vi "ReportPart.vi"(6 "试验项目":enum32{"手柄锁紧力", "手柄开启力", "手柄推拉力", "手柄保持力"}(ring), 8 "error in":errorcluster, 9 "索引IN":i32, 10 "合格":T1, 11 "report in":refnum<class "NI_report.lvclass">) -> (0 "error out 2":errorcluster caption="error out", 2 "索引OUT":i32, 3 "report out":refnum<class "NI_report.lvclass">)   [LabVIEW 2020]
uses:
  <vilib>/Utility/NIReport.llb/NI_report.lvclass
  OK.ctl
  <vilib>/Utility/NIReport.llb/image depth.ctl
  <vilib>/addons/_office/_exclsub.llb/font.ctl
  Global_Variable/A180648.vi
  <vilib>/Utility/NIReport.llb/Append Report Text (str wrap).vi
  Global_Variable/Global.vi
  <vilib>/addons/_office/word.llb/Word Easy Table (str).vi
  <vilib>/Utility/NIReport.llb/NI_ReportGenerationCore.lvlib
  <vilib>/addons/_office/NI_ReportGenerationToolkit.lvlib
  <vilib>/Utility/NIReport.llb/Word/NI_Word.lvclass
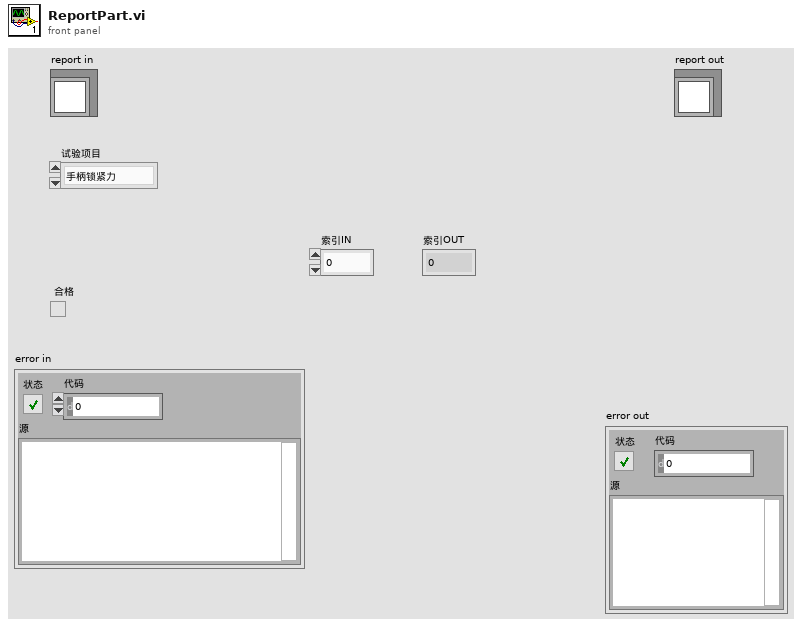
[diagram p1: front panel]
types:
  T1 = typedef "OK.ctl" = bool
  T2 = cluster{"Charset (-1)":i16, "Weight (-1)":i16, "Name":string, "Size":string}
  T3 = cluster{"Italic":enum16{"Italic Unchanged", "Italic On", "Italic Off"}, "Strike Through":enum16{"Strike Through Unchanged", "Strike Through On", "Strike Through Off"}, "Underline":enum16{"Underline Unchanged", "Underline On", "Underline Off"}, "Bold":enum16{"Bold Unchanged", "Bold On", "Bold Off"}}
  T4 = typedef "NI_ReportGenerationToolkit.lvlib/font.ctl" = cluster{"font name":string, "font size":dbl, "bold":u16, "italic":u16, "underline":u16, "strike through":u16, "font color":u32}
  T5 = typedef "NI_ReportGenerationCore.lvlib/image depth.ctl" = u16
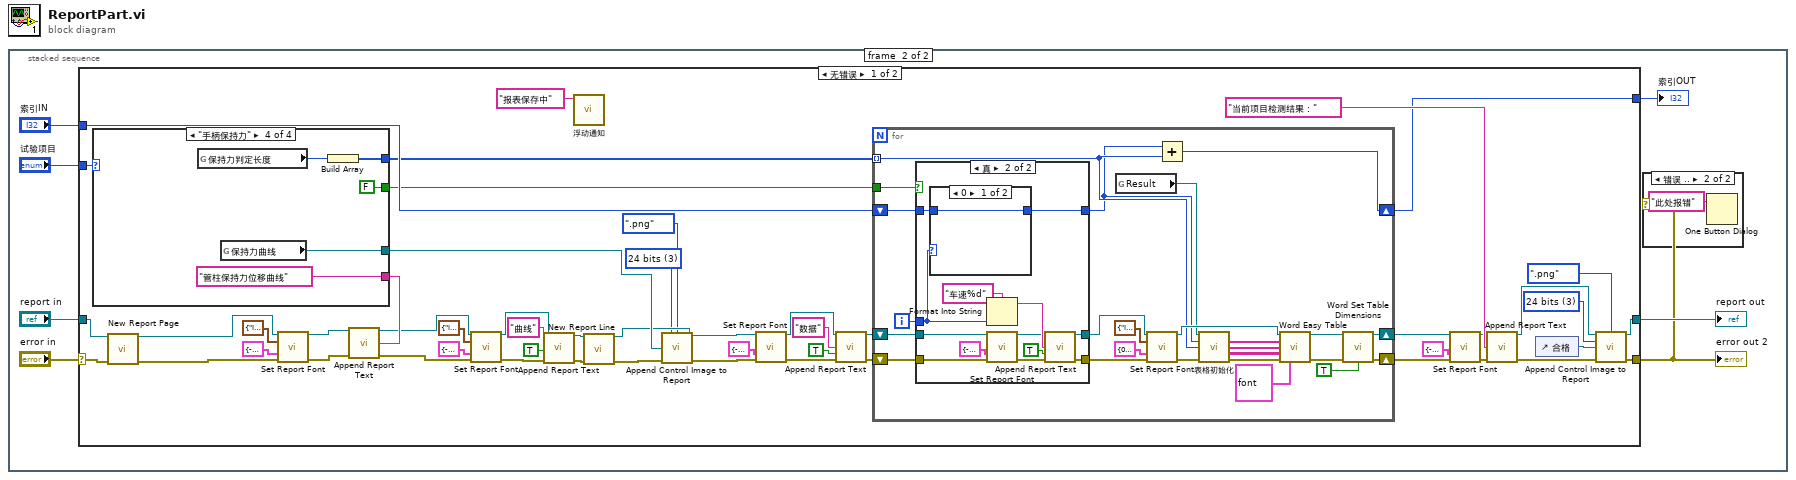
[diagram p0: block diagram]
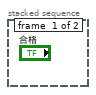
[diagram p2: hidden frame]
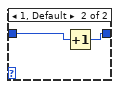
[diagram p5: hidden frame]
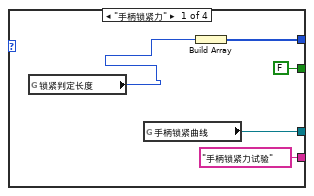
[diagram p6: hidden frame]
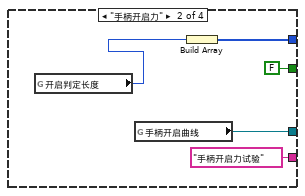
[diagram p7: hidden frame]
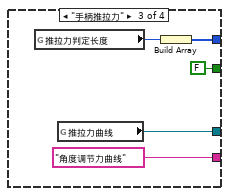
[diagram p8: hidden frame]
diagram:
  n1 = stacked-sequence {
    frame #0 {
    }
    frame #1 {
      n2 = case shown="无错误" "error in" {
        selector: "error in" -> [w53 w127]
        tunnel: [w48 w127] -> w1
        tunnel: "索引IN" -> [w20 w126]
        tunnel: "试验项目" -> [w23 _]
        tunnel: [w17 w126] -> w4
        tunnel: [w22 w125] -> w3
        tunnel: "report in" -> [w21 w125]
        frame No Error {
          w36 = T5 3 items=["B&W", "4 bits", "8 bits", "24 bits"] ("image depth")
          w46 = T5 3 items=["B&W", "4 bits", "8 bits", "24 bits"] ("image depth")
          n3 = case shown="\"手柄保持力\"" w23 {
            tunnel: [w109 w114 w119 w124] -> w39
            tunnel: ["手柄锁紧力试验" ("text") "手柄开启力试验" ("text") "角度调节力曲线" ("text") "管柱保持力位移曲线" ("text")] -> w57
            tunnel: [w107 w112 w115 w120] -> w19
            tunnel: [FALSE FALSE FALSE FALSE] -> w16
            frame "手柄锁紧力" {
              n4 = global read "判定参数.vi" "锁紧判定长度"() -> (w105:i32)
              n5 = global read "A180648.vi" "手柄锁紧曲线"() -> (w109:refnum<vi>)
              n6 = Build Array(w105) -> (w107:i32[])
            }
            frame "手柄开启力" {
              n7 = global read "判定参数.vi" "开启判定长度"() -> (w110:i32)
              n8 = global read "A180648.vi" "手柄开启曲线"() -> (w114:refnum<vi>)
              n9 = Build Array(w110) -> (w112:i32[])
            }
            frame "手柄推拉力" {
              n10 = global read "判定参数.vi" "推拉力判定长度"() -> (w117:i32)
              n11 = global read "A180648.vi" "推拉力曲线"() -> (w119:refnum<vi>)
              n12 = Build Array(w117) -> (w115:i32[])
            }
            frame "手柄保持力" {
              n13 = global read "判定参数.vi" "保持力判定长度"() -> (w122:i32)
              n14 = global read "A180648.vi" "保持力曲线"() -> (w124:refnum<vi>)
              n15 = Build Array(w122) -> (w120:i32[])
            }
          }
          n16 = call-dynamic "New Report Page.vi"("report in"=w21, "error in (no error)"=w53) -> ("report out"=w51:refnum<class "NI_report.lvclass">, "error out"=w52:errorcluster)  [unwired: 12 in]
          n17 = call-dynamic "Set Report Font.vi"("report in"=w51, "text options"=T3 {"Italic"=enum."Italic Unchanged", "Strike Through"=enum."Strike Through Unchanged", "Underline"=enum."Underline Unchanged", "Bold"=enum."Bold On"}, "font settings"=T2 {"Charset (-1)"=-1, "Weight (-1)"=-1, "Name"="楷体", "Size"="16 "}, "error in (no error)"=w52) -> ("report out"=w60:refnum<class "NI_report.lvclass">, "error out"=w59:errorcluster)  [unwired: 9 in, 1 out]
          n18 = call-poly <vilib>:"Append Report Text.vi"("report in"=w60, "text"=w57, "error in (no error)"=w59) -> ("report out"=w55:refnum<class "NI_report.lvclass">, "error out"=w54:errorcluster)  [unwired: 9 in, 2 out]
          n19 = call-dynamic "Set Report Font.vi"("report in"=w55, "text options"=T3 {"Italic"=enum."Italic Unchanged", "Strike Through"=enum."Strike Through Unchanged", "Underline"=enum."Underline Unchanged", "Bold"=enum."Bold Off"}, "font settings"=T2 {"Charset (-1)"=-1, "Weight (-1)"=-1, "Name"="宋体", "Size"="12"}, "error in (no error)"=w54) -> ("report out"=w30:refnum<class "NI_report.lvclass">, "error out"=w27:errorcluster)  [unwired: 9 in, 1 out]
          n20 = call-poly <vilib>:"Append Report Text.vi"("report in"=w30, "text"="曲线", "append on new line? (F)"=TRUE, "error in (no error)"=w27) -> ("report out"=w29:refnum<class "NI_report.lvclass">, "error out"=w28:errorcluster)  [unwired: 8 in, 2 out]
          n21 = call "浮动通知.vi"("通知内容"="报表保存中") -> ()  [unwired: 11 in]
          n22 = call-dynamic "New Report Line.vi"("report in"=w29, "error in (no error)"=w28) -> ("report out"=w37:refnum<class "NI_report.lvclass">, "error out"=w38:errorcluster)  [unwired: 12 in]
          n23 = call-dynamic "Append Control Image to Report.vi"("report in"=w37, "image file type (.jpg)"=enum16{".jpg", ".png"}.".png", "image depth"=w36, "ctrl reference"=w39, "error in (no error)"=w38) -> ("report out"=w34:refnum<class "NI_report.lvclass">, "error out"=w33:errorcluster)  [unwired: 7 in, 2 out]
          n24 = call-dynamic "Set Report Font.vi"("report in"=w34, "font settings"=T2 {"Charset (-1)"=-1, "Weight (-1)"=-1, "Name"="微软雅黑", "Size"="12 "}, "error in (no error)"=w33) -> ("report out"=w15:refnum<class "NI_report.lvclass">, "error out"=w12:errorcluster)  [unwired: 10 in, 1 out]
          n25 = call-poly <vilib>:"Append Report Text.vi"("report in"=w15, "text"="数据", "append on new line? (F)"=TRUE, "error in (no error)"=w12) -> ("report out"=w11:refnum<class "NI_report.lvclass">, "error out"=w10:errorcluster)  [unwired: 8 in, 2 out]
          n26 = for {
            tunnel: w19 -> [w70] mode=indexing
            shift-right: [w85] -> w41
            shift-left: w11 -> [w68]
            shift-right: [w84] -> w40
            shift-left: w10 -> [w67]
            shift-right: [w69] -> w17
            shift-left: w20 -> [w62]
            tunnel: w16 -> [w63]
            i -> [w64]
            n27 = case shown="真" w63 {
              tunnel: w68 -> [w88 w95]
              tunnel: w67 -> [w87 w94]
              tunnel: [w88 w93] -> w66
              tunnel: [w87 w92] -> w65
              tunnel: w64 -> [_ w89]
              tunnel: w62 -> [w86 w91]
              tunnel: [w86 w90] -> w61
              frame False {
              }
              frame True {
                n28 = case shown="0" w89 {
                  tunnel: [w102 w103] -> w90
                  tunnel: w91 -> [w102 w104]
                  frame 0 {
                  }
                  frame 1, Default {
                    n29 = Increment(x=w104) -> (x+1=w103:i32)
                  }
                }
                n30 = Format Into String(format string="车速%d" ("格式字符串"), w89) -> (resulting string=w101:string)  [unwired: 2 in, 1 out]
                n31 = call-dynamic "Set Report Font.vi"("report in"=w95, "font settings"=T2 {"Charset (-1)"=-1, "Weight (-1)"=-1, "Name"="宋体", "Size"="12 "}, "error in (no error)"=w94) -> ("report out"=w100:refnum<class "NI_report.lvclass">, "error out"=w99:errorcluster)  [unwired: 10 in, 1 out]
                n32 = call-poly <vilib>:"Append Report Text.vi"("report in"=w100, "text"=w101, "append on new line? (F)"=TRUE, "error in (no error)"=w99) -> ("report out"=w93:refnum<class "NI_report.lvclass">, "error out"=w92:errorcluster)  [unwired: 8 in, 2 out]
              }
            }
            n33 = global read "Global.vi" "Result"() -> (w71:refnum<vi>)
            n34 = call-dynamic "Set Report Font.vi"("report in"=w66, "text options"=T3 {"Italic"=enum."Italic Unchanged", "Strike Through"=enum."Strike Through Unchanged", "Underline"=enum."Underline Unchanged", "Bold"=enum."Bold Unchanged"}, "font settings"=T2 {"Charset (-1)"=0, "Weight (-1)"=-1, "Name"="微软雅黑", "Size"="12 "}, "error in (no error)"=w65) -> ("report out"=w73:refnum<class "NI_report.lvclass">, "error out"=w72:errorcluster)  [unwired: 9 in, 1 out]
            n35 = Add(x=w61, y=w70) -> (x+y=w69:i32)
            n36 = call "表格初始化.vi"("表格引用"=w71, "索引"=w61, "长度"=w70, "错误输入（无错误）"=w72) -> ("行首字符串[]"=w75:string[], "列首字符串[]"=w74:string[], "文本数据"=w77:string[][], "错误输出"=w80:errorcluster)  [unwired: 7 in, 1 out]
            n37 = call-poly <vilib>:"Word Easy Table.vi"("report in"=w73, "row headers"=w75, "column headers"=w74, "data"=w77, "error in (no error)"=w80, "font"=T4 {"font name"="宋体", "font size"=12.0, "bold"=2, "italic"=2, "underline"=2, "strike through"=2, "font color"=16777216}) -> ("report out"=w78:refnum<class "NI_report.lvclass">, "error out"=w79:errorcluster)  [unwired: 7 in, 1 out]
            n38 = call <vilib>:"Word Set Table Dimensions.vi"("report in"=w78, "error in (no error)"=w79, "fit to page width? (F)"=TRUE) -> ("report out"=w85:refnum<class "NI_report.lvclass">, "error out"=w84:errorcluster)  [unwired: 11 in]
          }
          n39 = call-dynamic "Set Report Font.vi"("report in"=w41, "font settings"=T2 {"Charset (-1)"=-1, "Weight (-1)"=-1, "Name"="宋体", "Size"="16 "}, "error in (no error)"=w40) -> ("report out"=w44:refnum<class "NI_report.lvclass">, "error out"=w45:errorcluster)  [unwired: 10 in, 1 out]
          n40 = call-poly <vilib>:"Append Report Text.vi"("report in"=w44, "text"="当前项目检测结果：", "error in (no error)"=w45) -> ("report out"=w50:refnum<class "NI_report.lvclass">, "error out"=w49:errorcluster)  [unwired: 9 in, 2 out]
          n41 = control-ref of="合格"() -> (w18:refnum<vi>)
          n42 = call-dynamic "Append Control Image to Report.vi"("report in"=w50, "image file type (.jpg)"=enum16{".jpg", ".png"}.".png", "image depth"=w46, "ctrl reference"=w18, "error in (no error)"=w49) -> ("report out"=w22:refnum<class "NI_report.lvclass">, "error out"=w48:errorcluster)  [unwired: 7 in, 2 out]
        }
        frame Error {
        }
      }
      "error out 2" <- w1
      "索引OUT" <- w4
      "report out" <- w3
      n43 = case shown="错误 .." w1 {
        frame No Error {
        }
        frame Error {
          n44 = One Button Dialog(message="此处报错" ("消息")) -> ()  [unwired: 1 in, 1 out]
        }
      }
    }
  }
